vi "Set Period.vi"(6 "Worker Alias":string="Message Pump", 7 "Caller":refnum<class "Worker.lvclass">, 8 "error in":errorcluster, 10 "Period (ms)":i32=-1) -> (0 "error out":errorcluster, 5 "dup Caller out":refnum<class "Worker.lvclass">)   [LabVIEW 2023, in "GUI.lvlib" / "Message Pump.lvclass"]
doc: "<b>Note: For ease of use, this VI is a wrapper around this Worker's standard Public API VIs. You can also use this Worker's Public API VIs in its place.</b>\n\nSets the wait time in milliseconds between pumped messages. 20 ms is the minimum possible wait time. A value of -1 will stop messages from being pumped.\n\nThis VI returns an error if the Message Pump Worker, as identified through <b>Worker Alias</b> is not found to exist.\n\n-----------\n\n<b>Inputs ></b>\n\n<b>Period (ms)</b>: The wait time in milliseconds between pumped messages. 20 ms is the minimum possible wait time. A value of -1 will stop messages from being pumped.\n\n<b>Worker Alias</b>: The name of the message pump. This name is local to the Worker it is called from. This input is required if multiple Message Pumps are to be used by the calling Worker."
uses:
  Message Pump.lvclass
  <vilib>/addons/_Workers/Library/Classes/Worker/Worker.lvclass
  rqp_Set EHL Timeout.ctl
  <vilib>/Utility/error.llb/Error Cluster From Error Code.vi
  <vilib>/ErrorRing/Error Ring.xnode
  Message Pump.lvclass/Message Pump.ctl
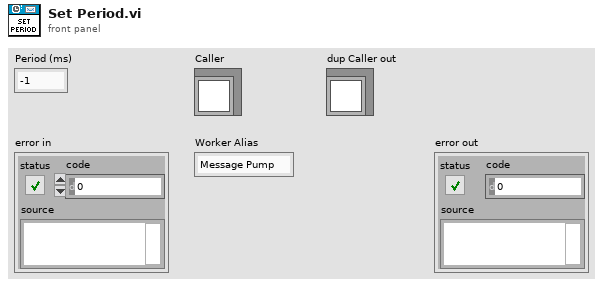
[diagram p1: front panel]
types:
  T1 = typedef "GUI.lvlib/Message Pump.lvclass/rqp_Set EHL Timeout.ctl" = cluster{"Timeout (ms)":i32}
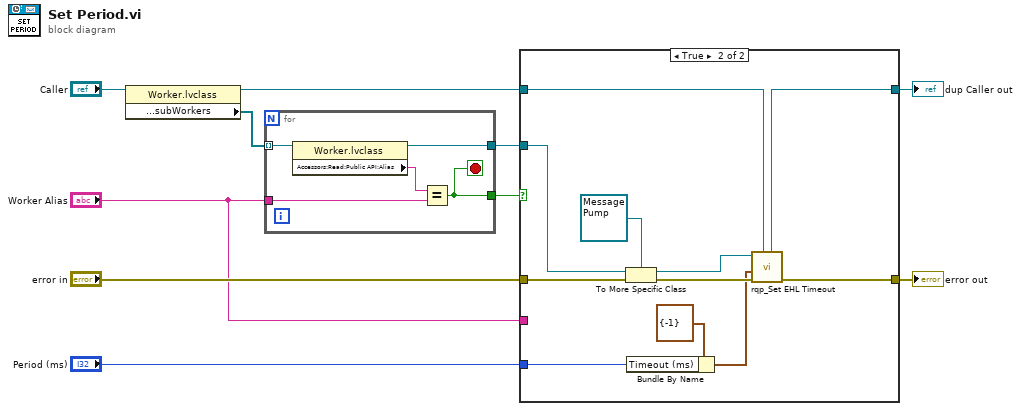
[diagram p0: block diagram]
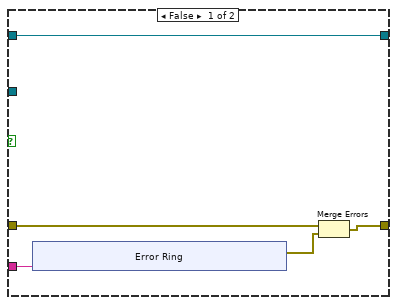
[diagram p2: hidden frame]
diagram:
  n1 = property class="Worker.lvclass"(reference="Caller") -> (reference out=w8:refnum<class "Worker.lvclass">, "Accessors:Read:Public API:subWorkers"=w7:refnum<class "Worker.lvclass">[])  [unwired: 1 in, 1 out]
  n2 = for {
    tunnel: w7 -> [w15] mode=indexing
    tunnel: "Worker Alias" -> [w13]
    tunnel: [w12] -> w5
    tunnel: [w11] -> w4
    stop <- w11 stop-if-true
    n3 = property class="Worker.lvclass"(reference=w15) -> (reference out=w12:refnum<class "Worker.lvclass">, "Accessors:Read:Public API:Alias"=w14:string)  [unwired: 1 in, 1 out]
    n4 = Equal?(x=w14, y=w13) -> (x = y?=w11:bool)
  }
  n5 = case shown="True" w4 {
    tunnel: [w17 w38] -> w9
    tunnel: w8 -> [w17 w37]
    tunnel: "error in" -> [w20 w36]
    tunnel: w5 -> [_ w34]
    tunnel: [w18 w31] -> w3
    tunnel: "Period (ms)" -> [_ w28]
    tunnel: "Worker Alias" -> [w16 _]
    frame False {
      n6 = xnode "Error Ring"("parameter 0"=w16) -> ("error out"=w19:errorcluster)
      n7 = Merge Errors(w20, w19) -> (w18:errorcluster)
    }
    frame True {
      n8 = To More Specific Class(target class=refnum<class "Message Pump.lvclass"> refnum ("_Message Pump"), reference=w34, error in=w36) -> (specific class reference=w32:refnum<class "Message Pump.lvclass">, error out=w35:errorcluster)
      n9 = Bundle By Name(cluster=T1 {"Timeout (ms)"=-1} ("Data in"), "Timeout (ms)"=w28) -> (w29:T1)
      n10 = call "rqp_Set EHL Timeout.vi"("Caller in"=w37, "error in"=w35, "Data in"=w29, "Message Pump in"=w32) -> ("error out"=w31:errorcluster, "dup Caller out"=w38:refnum<class "Worker.lvclass">)  [unwired: 5 in, 1 out]
    }
  }
  "error out" <- w3
  "dup Caller out" <- w9
